vi "ex5.vi"() -> ()   [LabVIEW 2019]
panel:
  out "deleted portion":dbl[][](array[numeric])
  out "size(s)":i32[](array[numeric])
  out "array w/ subset deleted 2":dbl[][](array[numeric])
  in  "index (row)":i32
  in  "length":i32
  in  "array":dbl[][](array[numeric])
  out "output array 2":dbl[](array[numeric])
  in  "new element/subarray 2":dbl
  in  "index 2":i32
  in  "new element/subarray":dbl
  in  "index":i32
  out "output array":dbl[](array[numeric])
  out "Waveform Graph":i32[](graph)
  in  "Array 2":i32[](array[numeric])
  out "valeur moyenne":dbl
  out "array décroissant":dbl[](array[numeric])
  out "min index(es)":i32
  out "min value":dbl
  out "max index(es)":i32
  out "max value":dbl
  out "array croissant":dbl[](array[numeric])
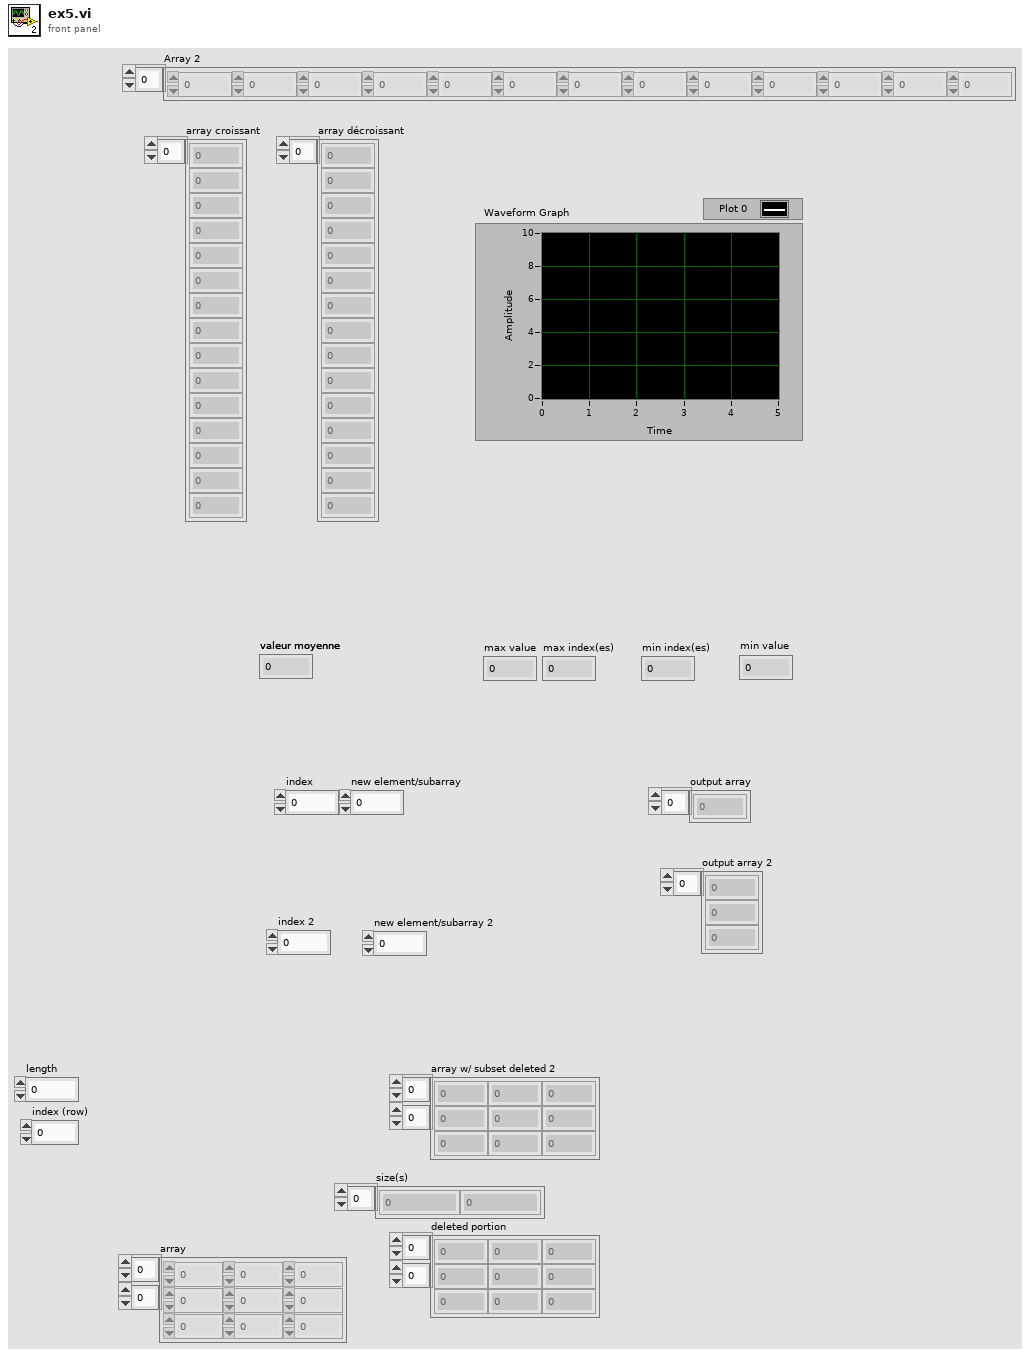
[diagram p1: front panel]
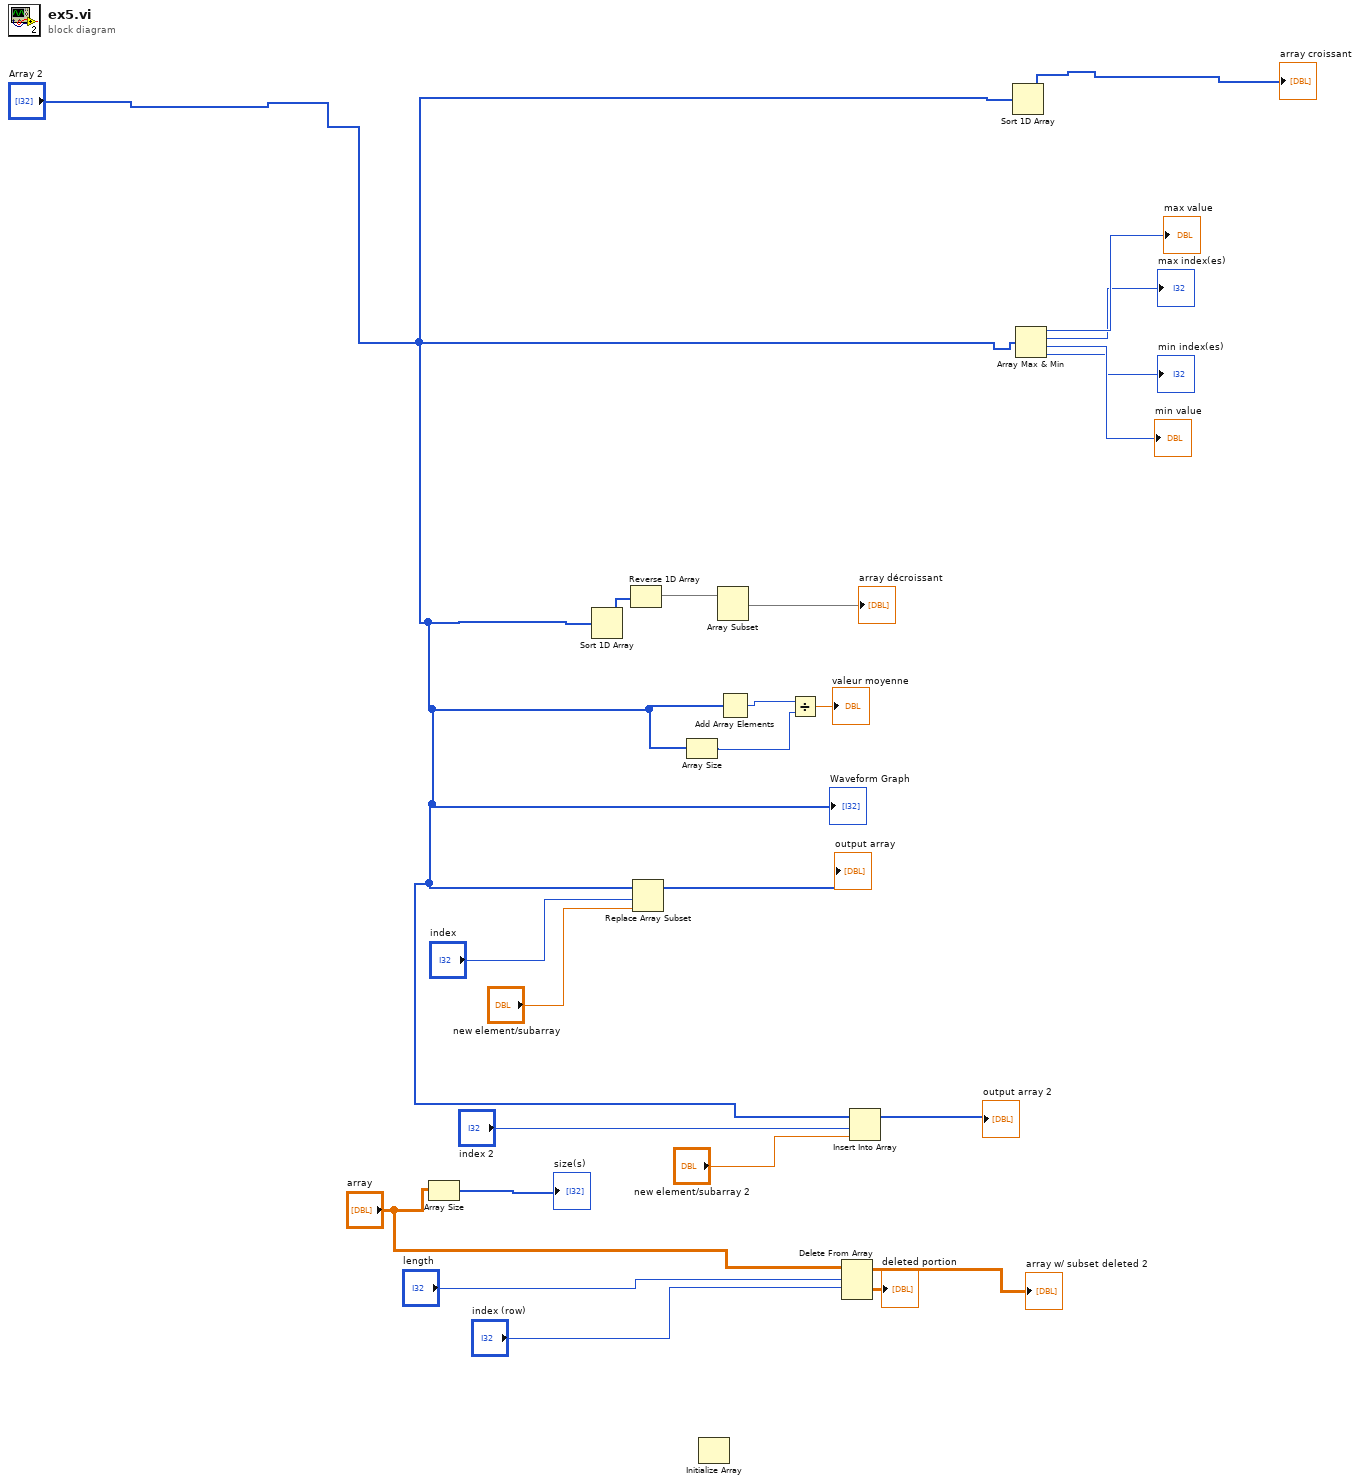
[diagram p0: block diagram]
diagram:
  n1 = Array Size(array="array") -> (size(s)=→"size(s)":i32[])
  n2 = Sort 1D Array(array="Array 2") -> (sorted array=w20:i32[])
  n3 = Reverse 1D Array(array=w20) -> (reversed array=w18:i32[])
  n4 = Replace Array Subset(array="Array 2", new element="new element/subarray", index="index") -> (→"output array":i32[])
  n5 = Array Size(array="Array 2") -> (size(s)=w14:i32)
  n6 = Initialize Array() -> ()  [unwired: 2 in, 1 out]
  n7 = Array Subset(array=w18) -> (→"array décroissant":i32[])  [unwired: 2 in]
  n8 = Add Array Elements(numeric array="Array 2") -> (sum=w16:i32)
  n9 = Divide(x=w16, y=w14) -> (x/y=→"valeur moyenne":dbl)
  n10 = Delete From Array(array="array", length="length", index (row)="index (row)") -> (deleted portion=→"deleted portion":dbl[][], array with subset deleted=→"array w/ subset deleted 2":dbl[][])  [unwired: 1 in]
  n11 = Insert Into Array(array="Array 2", index="index 2", new element="new element/subarray 2") -> (→"output array 2":i32[])
  n12 = Sort 1D Array(array="Array 2") -> (sorted array=→"array croissant":i32[])
  n13 = Array Max & Min(array="Array 2") -> (max value=→"max value":i32, max index (indices)=→"max index(es)":i32, min value=→"min value":i32, min index (indices)=→"min index(es)":i32)
  "Waveform Graph" <- "Array 2"
